vi "central difference (dbl).vi"(3 "Y":dbl[](array[numeric]), 4 "pad":bool=TRUE) -> (5 "0.5*(Y(i+1)-Y(i-1))":dbl[](array[numeric]))   [LabVIEW 2010, in "common.lvlib"]
uses:
  common.lvlib
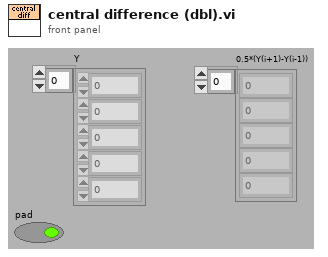
[diagram p1: front panel]
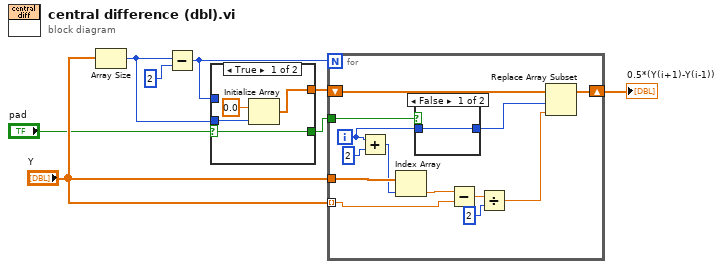
[diagram p0: block diagram]
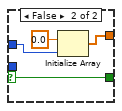
[diagram p2: hidden frame]
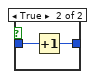
[diagram p3: hidden frame]
diagram:
  n1 = Array Size(array="Y") -> (size(s)=w4:i32)
  n2 = Subtract(x=w4, y=2 ("size(s)")) -> (x-y=w5:i32)
  n3 = case shown="True" "pad" {
    selector: "pad" -> [w9 w13]
    tunnel: w5 -> [_ w14]
    tunnel: w4 -> [w12 _]
    tunnel: [w10 w15] -> w3
    tunnel: [w9 w13] -> w2
    frame True {
      n4 = Initialize Array(0.0 ("element"), w12) -> (w10:dbl[])
    }
    frame False {
      n5 = Initialize Array(0.0 ("element"), w14) -> (w15:dbl[])
    }
  }
  n6 = for {
    N: w5 -> [_]
    tunnel: "Y" -> [w29]
    shift-right: [w25] -> w1
    shift-left: w3 -> [w26]
    tunnel: "Y" -> [w18] mode=indexing
    tunnel: w2 -> [w17]
    i -> [w24]
    n7 = Add(x=w24, y=2 ("size(s)")) -> (x+y=w28:i32)
    n8 = Index Array(array=w29, index=w28) -> (element=w27:dbl)
    n9 = case shown="False" w17 {
      tunnel: w24 -> [w30 w32]
      tunnel: [w30 w31] -> w19
      frame False {
      }
      frame True {
        n10 = Increment(x=w32) -> (x+1=w31:i32)
      }
    }
    n11 = Subtract(x=w27, y=w18) -> (x-y=w22:dbl)
    n12 = Divide(x=w22, y=2 ("size(s)")) -> (x/y=w20:dbl)
    n13 = Replace Array Subset(array=w26, new element=w20, index=w19) -> (w25:dbl[])
  }
  "0.5*(Y(i+1)-Y(i-1))" <- w1
